vi "get number of scans per acquisition.vi"(8 "error in (no error)":errorcluster, 11 "LineCCD in":refnum<class "LineCCD.lvclass">) -> (0 "error out":errorcluster, 3 "LineCCD out":refnum<class "LineCCD.lvclass">)   [LabVIEW 2012, in "LineCCD.lvclass"]
uses:
  LineCCD.lvclass
  <instrlib>/ALPHALAS CCD S Series/ALPHALAS CCD S Series.lvlib
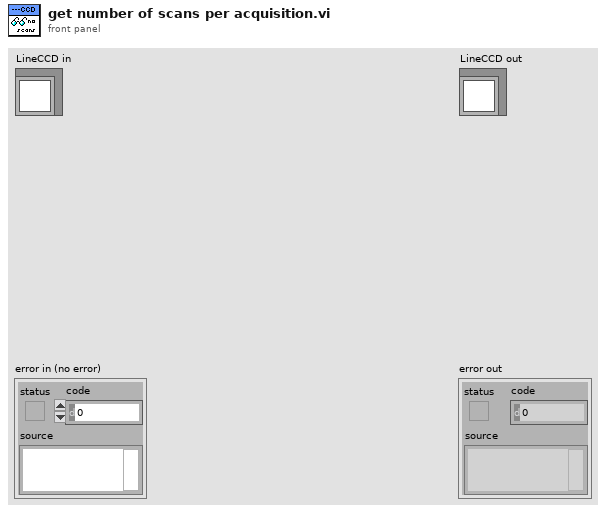
[diagram p1: front panel]
types:
  T1 = typedef "ALPHALAS CCD S Series.lvlib/Scans per Acquisition.ctl" = u32
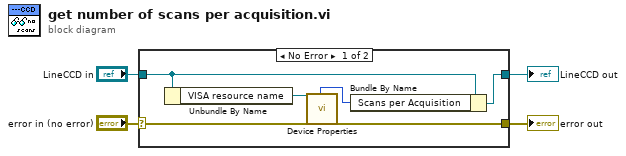
[diagram p0: block diagram]
diagram:
  n1 = case shown="No Error" "error in (no error)" {
    selector: "error in (no error)" -> [w9 w12]
    tunnel: [w8 w12] -> w3
    tunnel: [w5 w11] -> w1
    tunnel: "LineCCD in" -> [w6 w11]
    frame No Error {
      n2 = Unbundle By Name(w6) -> ("VISA resource name"=w10:refnum<visa-resource-name>)
      n3 = call <instrlib>:"Device Properties.vi"("VISA resource name"=w10, "error in (no error)"=w9) -> ("Scans per Acquisition"=w7:T1, "error out"=w8:errorcluster)  [unwired: 6 in, 18 out]
      n4 = Bundle By Name(cluster=w6, "Scans per Acquisition"=w7) -> (w5:refnum<class "LineCCD.lvclass">)
    }
    frame Error {
    }
  }
  "error out" <- w3
  "LineCCD out" <- w1
